vi "Auto_Routine_Triangle.vi"   [LabVIEW 2020]
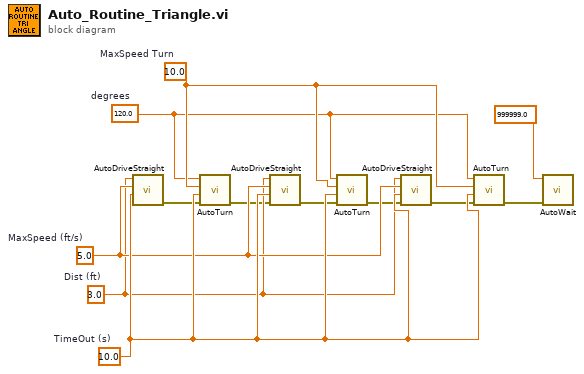
[diagram p0: block diagram]
diagram:
  w11 = 10.0  # TimeOut (s)
  w10 = 10.0  # MaxSpeed Turn
  w9 = 5.0  # MaxSpeed (ft/s)
  w8 = 120.0  # degrees
  w7 = 3.0  # Dist (ft)
  n1 = call "AutoDriveStraight.vi"("TimeOut (s)"=w11, "MaxSpeed (ft/s)"=w9, "Dist (ft)"=w7) -> ("error out"=w1:errorcluster)  [unwired: 8 in]
  n2 = call "AutoTurn.vi"("error in (no error)"=w1, "TimeOut (s)"=w11, "MaxSpeed (ft/s)"=w10, "degrees"=w8) -> ("error out"=w2:errorcluster)  [unwired: 7 in]
  n3 = call "AutoDriveStraight.vi"("error in (no error)"=w2, "TimeOut (s)"=w11, "MaxSpeed (ft/s)"=w9, "Dist (ft)"=w7) -> ("error out"=w3:errorcluster)  [unwired: 7 in]
  n4 = call "AutoTurn.vi"("error in (no error)"=w3, "TimeOut (s)"=w11, "MaxSpeed (ft/s)"=w10, "degrees"=w8) -> ("error out"=w4:errorcluster)  [unwired: 7 in]
  n5 = call "AutoDriveStraight.vi"("error in (no error)"=w4, "TimeOut (s)"=w11, "MaxSpeed (ft/s)"=w9, "Dist (ft)"=w7) -> ("error out"=w5:errorcluster)  [unwired: 7 in]
  n6 = call "AutoTurn.vi"("error in (no error)"=w5, "TimeOut (s)"=w11, "MaxSpeed (ft/s)"=w10, "degrees"=w8) -> ("error out"=w6:errorcluster)  [unwired: 7 in]
  n7 = call "AutoWait.vi"("error in (no error)"=w6, "TimeOut (s)"=999999.0) -> ()  [unwired: 9 in, 1 out]
